vi "teleop drive straight.vi"(2 "Reverse":bool, 3 "Speed":dbl) -> (0 "right":dbl, 1 "left":dbl)   [LabVIEW 2011]
uses:
  Robot Global Data.vi
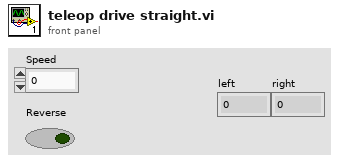
[diagram p1: front panel]
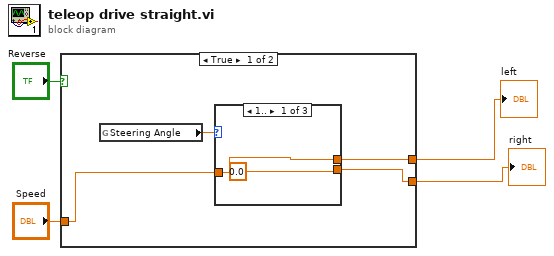
[diagram p0: block diagram]
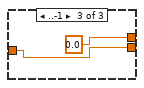
[diagram p3: hidden frame]
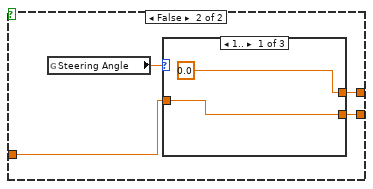
[diagram p4: hidden frame]
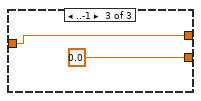
[diagram p6: hidden frame]
diagram:
  n1 = case shown="True" "Reverse" {
    tunnel: "Speed" -> [w5 w16]
    tunnel: [w7 w15] -> w2
    tunnel: [w6 w14] -> w1
    frame True {
      n2 = global read "Robot Global Data.vi" "Steering Angle"() -> (w8:dbl)
      n3 = case shown="1.." w8 {
        tunnel: w5 -> [w9 w11 w12]
        tunnel: [w9 w11 0.0 ("X axis value")] -> w7
        tunnel: [0.0 ("X axis value") w11 w12] -> w6
        frame 1.. {
        }
        frame Default {
        }
        frame ..-1 {
        }
      }
    }
    frame False {
      n4 = global read "Robot Global Data.vi" "Steering Angle"() -> (w17:dbl)
      n5 = case shown="1.." w17 {
        tunnel: w16 -> [w18 w20 w22]
        tunnel: [0.0 ("X axis value") w20 w22] -> w15
        tunnel: [w18 w20 0.0 ("Right axis value")] -> w14
        frame 1.. {
        }
        frame Default {
        }
        frame ..-1 {
        }
      }
    }
  }
  "left" <- w2
  "right" <- w1
